vi "DDSTestShiftReg.vi"() -> ()   [LabVIEW 2016]
panel:
  out "return count":u32=489
  in  "Duration [ms]":dbl[](array[numeric])=[1.0, 1.0, 1.0, 1.0, 1.0, 1.0]
  out "Write Instructions":string="interactive off\rdds reset\r\rdcp 1 spi:STP0=0x8E39051EB852\rdcp 1 spi:CFR2=0x1000080\rdcp update:u\rdcp 1 spi:STP0=0x3FFF000000418937\r\rdcp 1 wait:125000h:\r\rdcp update:u\rdcp 1 spi:STP0=0x418937\r\rdcp 1 wait:125000h:\r\rdcp update:u\rdcp 1 spi:STP0=0x3FFF000000418937\r\rdcp 1 wait:125000h:\r\rdcp update:u\rdcp 1 spi:STP0=0x418937\r\rdcp 1 wait:125000h:\r\rdcp update:u\rdcp 1 spi:STP0=0x3FFF000000418937\r\rdcp 1 wait:125000h:\r\rdcp update:u\rdcp 1 spi:STP0=0x418937\r\rdcp 1 wait:125000h:\r\rdcp update:u\rdcp start\r"
  in  "phase degrees (0..360) 2":dbl[](array[numeric])=[0.0, 0.0, 0.0, 0.0, 0.0, 0.0] format="%#_13g"
  in  "amplitude (0..1) 2":dbl[](array[numeric])=[1.0, 0.0, 1.0, 0.0, 1.0, 0.0] format="%#_13g"
  in  "frequency Hz (0..400M) 2":dbl[](array[numeric])=[1000000.0, 1000000.0, 1000000.0, 1000000.0, 1000000.0, 1000000.0] format="%#_13g"
  out "error out":errorcluster={"status"=TRUE, "code"=-1073807339, "source"="VISA Read in DDSTestShiftReg.vi"}
  out "Read buffer":string="Interactive off\r\nDDS reset OK (0, 0)\r\n"
  in  "FlexDDS-NG USB VISA resource name (COM)":refnum<visa-resource-name>="COM7"
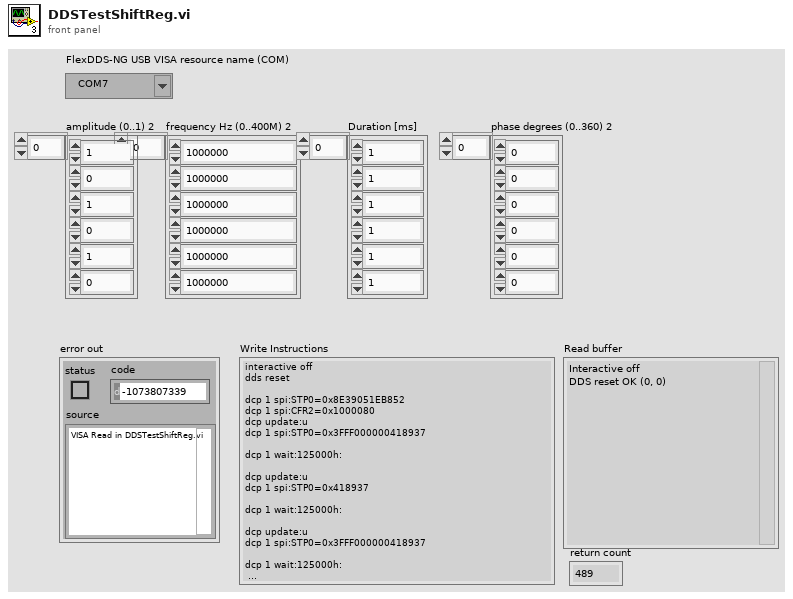
[diagram p1: front panel]
types:
  T1 = enum32{"Channel 0", "Channel 1", "Both channels"}
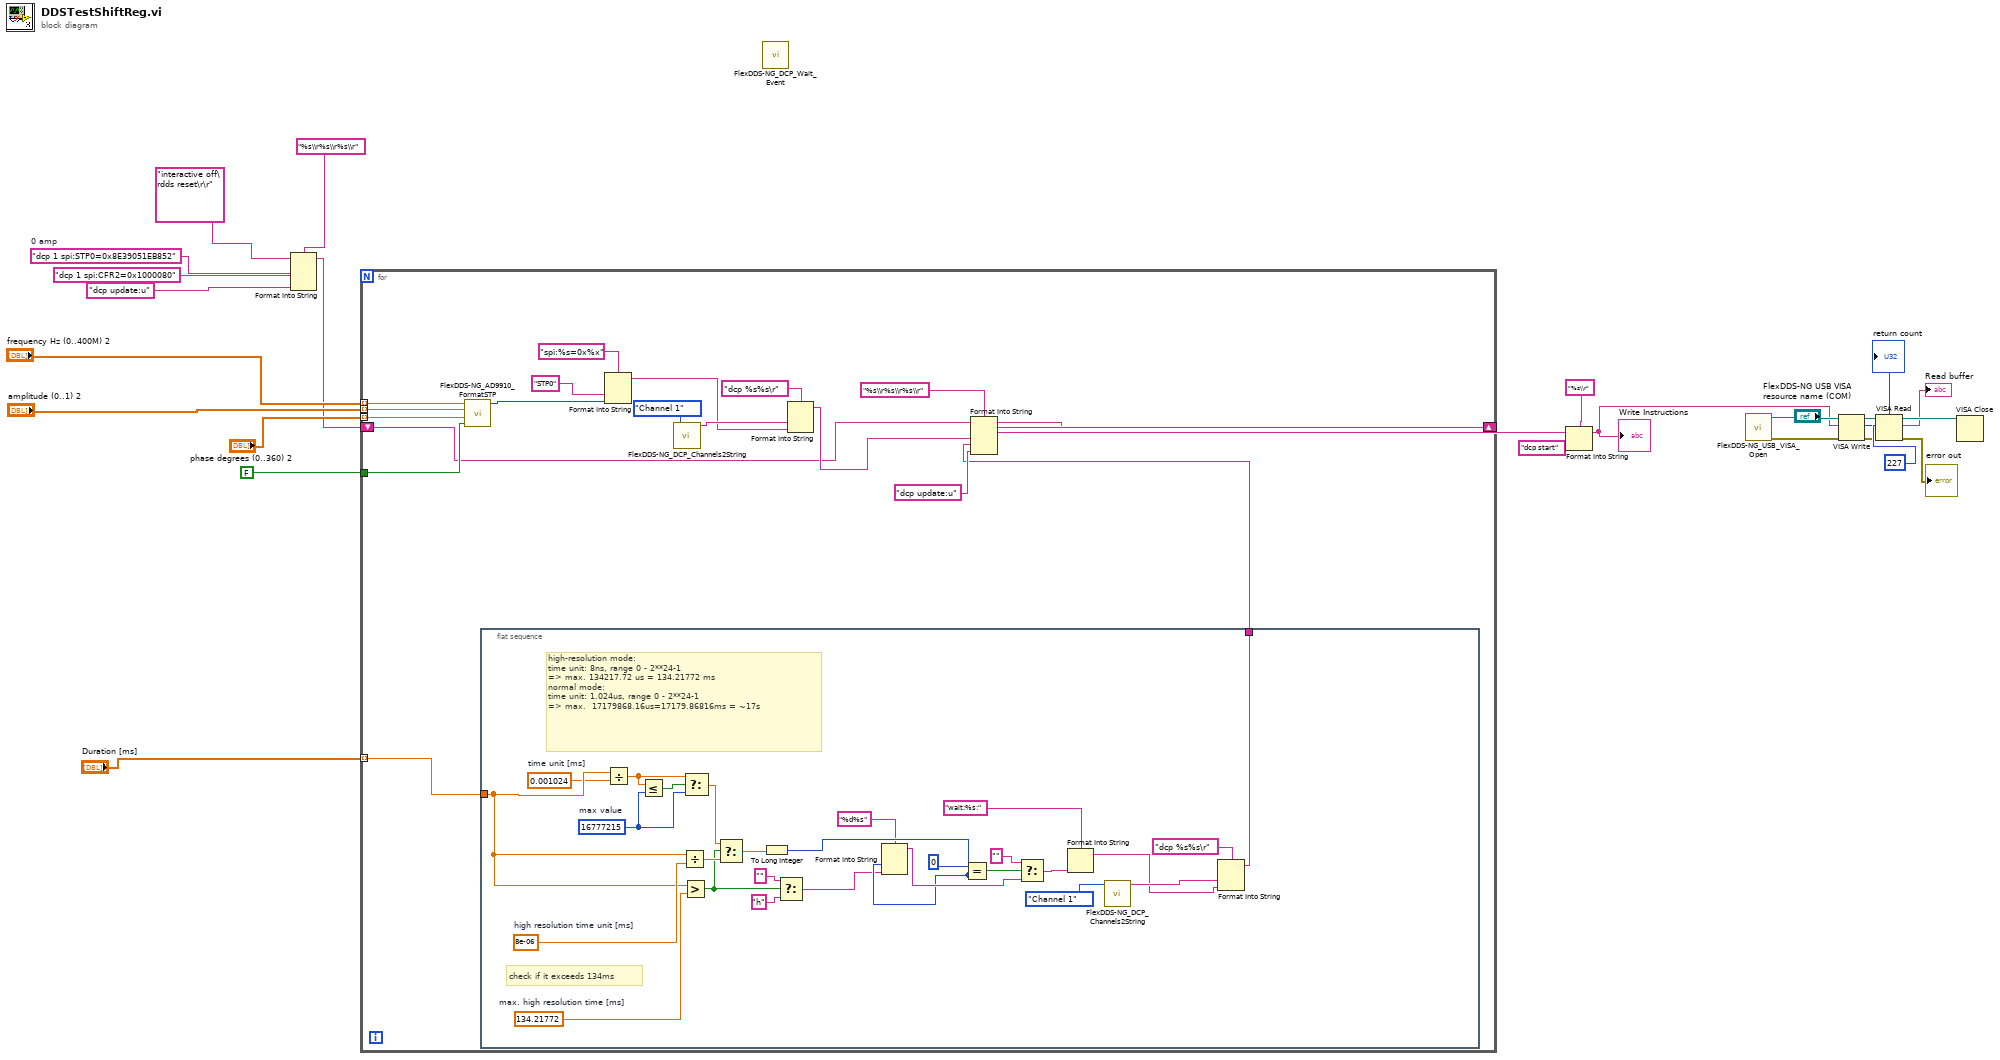
[diagram p0: block diagram]
diagram:
  w8 = "dcp 1 spi:STP0=0x8E39051EB852"  # 0 amp
  n1 = Format Into String(format string="%s\\r%s\\r%s\\r", initial string="interactive off\rdds reset\r\r" ("appended instruction string 3"), w8, "dcp 1 spi:CFR2=0x1000080", "dcp update:u" ("input 2")) -> (resulting string=w7:string)  [unwired: 1 in, 1 out]
  n2 = for {
    tunnel: "frequency Hz (0..400M) 2" -> [w43] mode=indexing
    tunnel: "amplitude (0..1) 2" -> [w42] mode=indexing
    tunnel: "phase degrees (0..360) 2" -> [w41] mode=indexing
    tunnel: FALSE ("mirror frequency?") -> [w40]
    shift-right: [w29] -> w4
    shift-left: w7 -> [w28]
    tunnel: "Duration [ms]" -> [w26] mode=indexing
    n3 = call "FlexDDS-NG_AD9910_FormatSTP.vi"("mirror frequency?"=w40, "phase degrees (0..360)"=w41, "amplitude (0..1)"=w42, "frequency Hz (0..400M)"=w43) -> ("single-tone profile (STP) out"=w37:u64)  [unwired: 4 in, 3 out]
    n4 = flat-sequence {
      tunnel: w26 -> [w64]
      tunnel: [w44] -> w27
      frame #0 {
        w68 = 16777215  # max value
        w63 = 0.001024  # time unit [ms]
        w65 = 8e-06  # high resolution time unit [ms]
        w61 = 134.21772  # max. high resolution time [ms]
        # "check if it exceeds 134ms"
        # "high-resolution mode:\ntime unit: 8ns, range 0 - 2**24-1\n=> max. 134217.72 us = 134.21772 ms\nnormal mode:\ntime unit: 1.024us, range 0 - 2**24-1\n=> max.  17179868.16us=17179.86816ms = ~17s"
        n5 = Divide(x=w64, y=w63) -> (x/y=w70:dbl)
        n6 = Less Or Equal?(x=w70, y=w68) -> (x <= y?=w67:bool)
        n7 = Divide(x=w64, y=w65) -> (x/y=w66:dbl)
        n8 = Greater?(x=w64, y=w61) -> (0:w60:bool)
        n9 = Select(t=w70, s=w67, f=w68) -> (s? t:f=w69:dbl)
        n10 = Select(t=w69, s=w60, f=w66) -> (s? t:f=w62:dbl)
        n11 = To Long Integer(number=w62) -> (32bit integer=w53:i32)
        n12 = Select(t="", s=w60, f="h") -> (s? t:f=w51:string)
        n13 = Format Into String(format string="%d%s", w53, w51) -> (resulting string=w57:string)  [unwired: 2 in, 1 out]
        n14 = Equal?(x=0, y=w53) -> (x = y?=w55:bool)
        n15 = Select(t="", s=w55, f=w57) -> (s? t:f=w49:string)
        n16 = Format Into String(format string="wait:%s:", w49) -> (resulting string=w45:string)  [unwired: 2 in, 1 out]
        n17 = call "FlexDDS-NG_DCP_Channels2String.vi"("Channels"=T1."Channel 1") -> ("channels string"=w46:string)  [unwired: 10 in]
        n18 = Format Into String(format string="dcp %s%s\r", w46, w45) -> (resulting string=w44:string)  [unwired: 2 in, 1 out]
      }
    }
    n19 = Format Into String(format string="spi:%s=0x%x", "STP0" ("AD9910 register name"), w37) -> (resulting string=w33:string)  [unwired: 2 in, 1 out]
    n20 = call "FlexDDS-NG_DCP_Channels2String.vi"("Channels"=T1."Channel 1" ("Channels 2")) -> ("channels string"=w34:string)  [unwired: 10 in]
    n21 = Format Into String(format string="dcp %s%s\r", w34, w33) -> (resulting string=w30:string)  [unwired: 2 in, 1 out]
    n22 = Format Into String(format string="%s\\r%s\\r%s\\r", initial string=w28, w30, w27, "dcp update:u" ("input 2")) -> (resulting string=w29:string)  [unwired: 1 in, 1 out]
  }
  n23 = call "FlexDDS-NG_DCP_Wait_Event.vi"() -> ()  [unwired: 11 in, 1 out]
  n24 = Format Into String(format string="%s\\r", initial string=w4, "dcp start" ("input 4")) -> (resulting string=w3:string)  [unwired: 1 in, 1 out]
  "Write Instructions" <- w3
  n25 = call "FlexDDS-NG_USB_VISA_Open.vi"("FlexDDS-NG USB VISA resource name (COM)"="FlexDDS-NG USB VISA resource name (COM)") -> ("error out"=w23:errorcluster, "FlexDDS-NG USB VISA resource name out"=w24:refnum<visa-resource-name>)  [unwired: 9 in]
  n26 = VISA Write(VISA resource name=w24, write buffer=w3, error in (no error)=w23) -> (VISA resource name out=w19:refnum<visa-resource-name>, return count=→"return count":u32, error out=w17:errorcluster)
  n27 = VISA Read(VISA resource name=w19, byte count=u32 227, error in (no error)=w17) -> (VISA resource name out=w22:refnum<visa-resource-name>, read buffer=→"Read buffer":string, error out=→"error out":errorcluster)  [unwired: 1 out]
  n28 = VISA Close(VISA resource name=w22) -> ()  [unwired: 1 in, 1 out]
